vi "SEW.vi"() -> ()   [LabVIEW 2018]
uses:
  <userlib>/PNIO/PNIO.dll
panel:
  in  "Acknowledge":bool
  out "data_write":u8[](array[numeric])
  out "Status":u16 format="%x"
  out "Cluster":T1
  out "NIST_A":u32
  out "ZSW1":u16 format="%x"
  in  "ON/OFF":bool
  in  "Speed setpoint":sgl format="%.2f rpm"
  in  "stop":bool
  out "data_read":u8[](array[numeric]) format="%x"
  in  "number_bytes":u32=32
  out "error_write":u32 format="%x"
  out "error_read":u32 format="%x"
  out "state":bool
  in  "output_adress":u32
  in  "input_adress":u32
  out "ErrorCode":u32
  in  "Path":path=path "C:/Users/Messknecht/Desktop/LabVIEW/sew_eurodrive/SEW_Vi/PROFINET Driver_1.PROFINET Driver.PNDriverConfiguration.xml"
  in  "mac_adress":string="f8:b1:56:9d:5d:4b"
  out "function return":u32 format="%x"
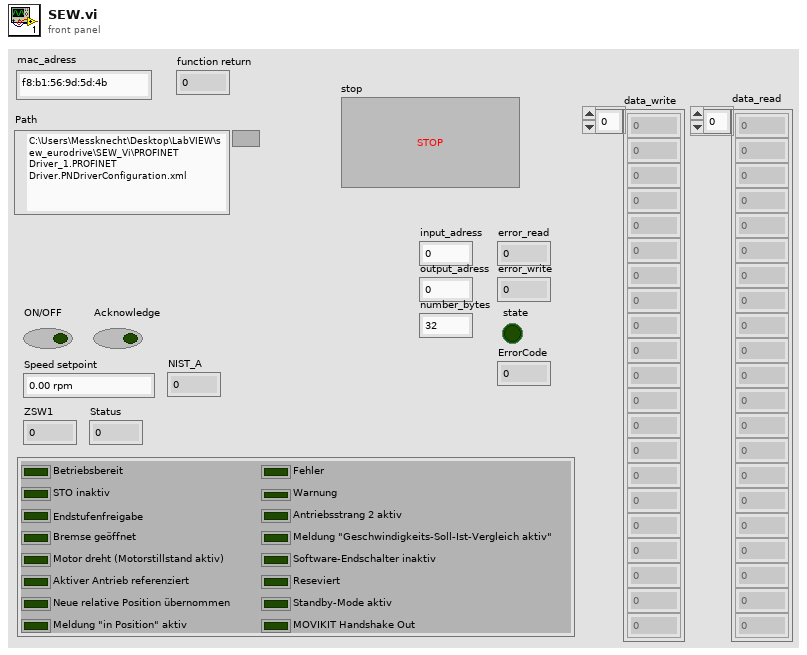
[diagram p1: front panel]
types:
  T1 = cluster{"Betriebsbereit":bool, "STO inaktiv":bool, "Endstufenfreigabe":bool, "Bremse geöffnet":bool, "Motor dreht (Motorstillstand aktiv)":bool, "Aktiver Antrieb referenziert":bool, "Neue relative Position übernommen":bool, "Meldung \"in Position\" aktiv":bool, "Fehler":bool, "Warnung":bool, "Antriebsstrang 2 aktiv":bool, "Meldung \"Geschwindigkeits-Soll-Ist-Vergleich aktiv\"":bool, "Software-Endschalter inaktiv":bool, "Reseviert":bool, "Standby-Mode aktiv":bool, "MOVIKIT Handshake Out":bool}
  T2 = cluster{"Boolean array[0]":bool, "Boolean array[1]":bool, "Boolean array[2]":bool, "Boolean array[3]":bool, "Boolean array[4]":bool, "Boolean array[5]":bool, "Boolean array[6]":bool, "Boolean array[7]":bool, "Boolean array[8]":bool, "Boolean array[9]":bool, "Boolean array[10]":bool, "Boolean array[11]":bool, "Boolean array[12]":bool, "Boolean array[13]":bool, "Boolean array[14]":bool, "Boolean array[15]":bool}
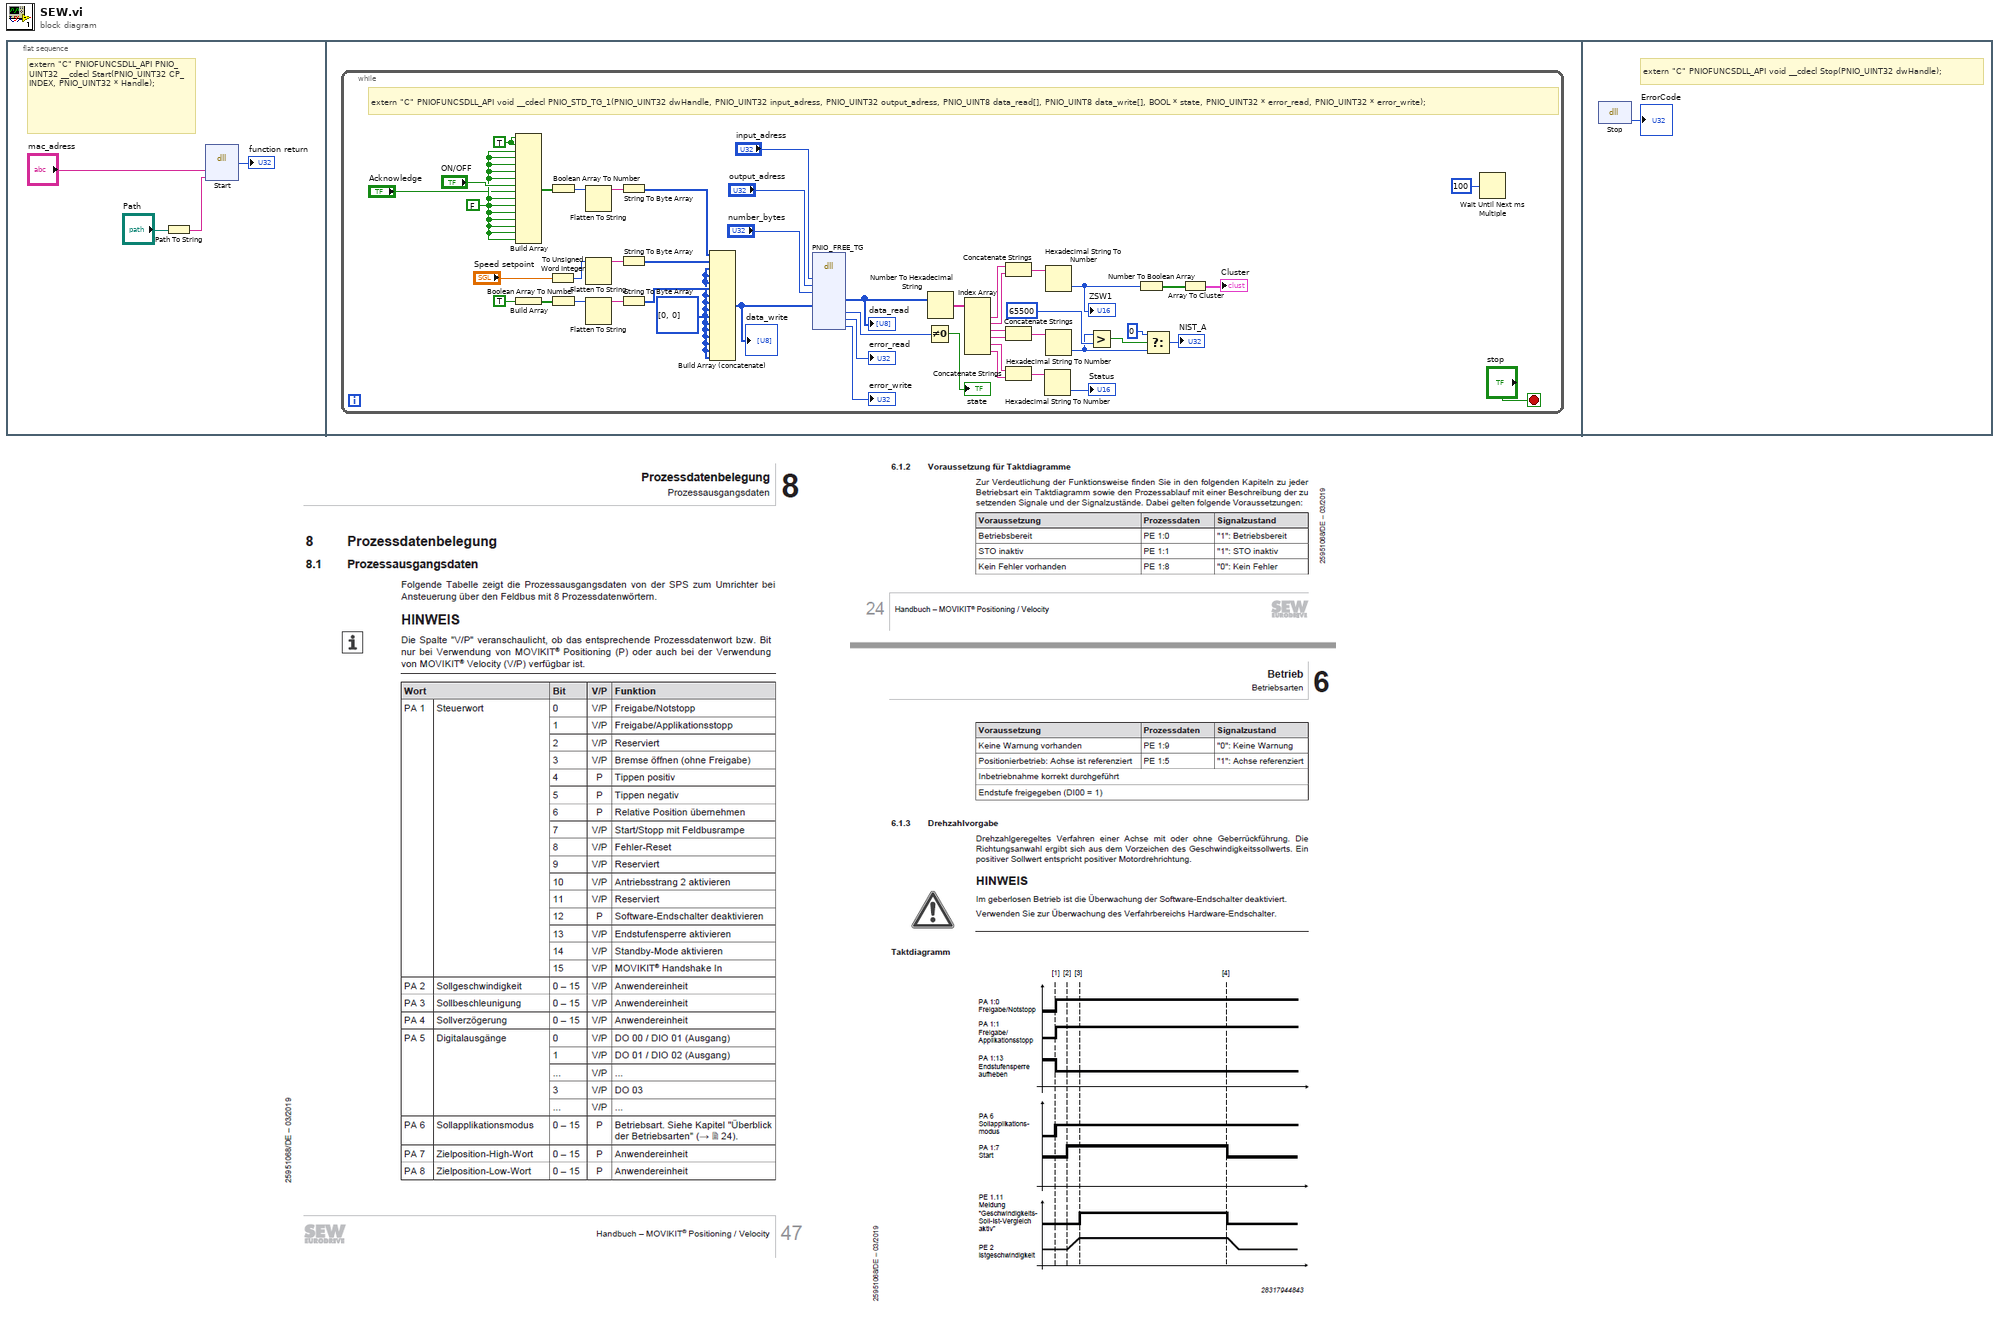
[diagram p0: block diagram]
diagram:
  n1 = flat-sequence {
    frame #0 {
      # "extern \"C\" PNIOFUNCSDLL_API PNIO_UINT32 __cdecl Start(PNIO_UINT32 CP_INDEX, PNIO_UINT32 * Handle);"
      n2 = Path To String(path="Path") -> (string=w1:string)
      n3 = dll-call lib="C:/Program Files (x86)/National Instruments/LabVIEW 2018/user.lib/PNIO/PNIO.dll" fn="Start"("mac_adress"="mac_adress", "xml_name"=w1) -> ("Rückgabetyp"=→"function return":u32)  [unwired: 5 in, 2 out]
    }
    frame #1 {
      n4 = while {
        stop <- "stop" stop-if-true
        w29 = u8[] [0, 0] ("unsigned byte array")
        w27 = FALSE
        w40 = TRUE
        # "extern \"C\" PNIOFUNCSDLL_API void __cdecl PNIO_STD_TG_1(PNIO_UINT32 dwHandle, PNIO_UINT32 input_adress, PNIO_UINT32 output_adress, PNIO_UINT8 data_read[], PNIO_UINT8 data_write[], BOOL * state, PNIO_UINT32 * error_read, PNIO_UINT32 * error_write);"
        n5 = Build Array(w40, w40, w27, w27, w27, w27, w27, "ON/OFF", "Acknowledge", w27, w27, w27, w27, w27, w27, w27) -> (w30:bool[])
        n6 = Build Array(TRUE) -> (w32:bool[])
        n7 = To Unsigned Word Integer(number="Speed setpoint") -> (unsigned 16bit integer=w39:u16)
        n8 = Boolean Array To Number ("Boolesches Array nach Zahl")(Boolean array=w30) -> (number=w41:u16)
        n9 = Boolean Array To Number ("Boolesches Array nach Zahl")(Boolean array=w32) -> (number=w33:u16)
        n10 = Flatten To String(anything=w41) -> (data string=w43:string)  [unwired: 3 in, 2 out]
        n11 = Flatten To String(anything=w39) -> (data string=w44:string)  [unwired: 3 in, 2 out]
        n12 = Flatten To String(anything=w33) -> (data string=w38:string)  [unwired: 3 in, 2 out]
        n13 = String To Byte Array(string=w43) -> (unsigned byte array=w42:u8[])
        n14 = String To Byte Array(string=w44) -> (unsigned byte array=w34:u8[])
        n15 = String To Byte Array(string=w38) -> (unsigned byte array=w37:u8[])
        n16 = Build Array (concatenate)(w42, w34, w29, w29, w29, w37, w29, w29, w29, w29, w29, w29, w29, w29, w29, w29) -> (w35:u8[])
        "data_write" <- w35
        n17 = dll-call lib="C:/Program Files (x86)/National Instruments/LabVIEW 2018/user.lib/PNIO/PNIO.*" fn="PNIO_FREE_TG"("input_adress"="input_adress", "output_adress"="output_adress", "number_bytes"="number_bytes", "data_write"=w35) -> ("data_read"=w25:u8[], "state"=w48:i32, "error_read"=→"error_read":u32, "error_write"=→"error_write":u32)  [unwired: 12 in, 2 out]
        "data_read" <- w25
        n18 = Not Equal To 0?(x=w48) -> (x != 0?=→"state":bool)
        n19 = Number To Hexadecimal String(2:w25) -> (0:w24:string[])  [unwired: 1 in]
        n20 = Index Array(array=w24) -> (element #1=w21:string, element #2=w20:string, element #3=w18:string, element #4=w17:string, element #5=w13:string, element #6=w12:string)  [unwired: 6 in]
        n21 = Concatenate Strings(w21, w20) -> (w19:string)
        n22 = Concatenate Strings(w18, w17) -> (w16:string)
        n23 = Concatenate Strings(w13, w12) -> (w15:string)
        n24 = Hexadecimal String To Number(string=w15) -> (number=→"Status":u32)  [unwired: 2 in, 1 out]
        n25 = Hexadecimal String To Number(string=w19) -> (number=w11:u32)  [unwired: 2 in, 1 out]
        "ZSW1" <- w11
        n26 = Hexadecimal String To Number(string=w16) -> (number=w7:u32)  [unwired: 2 in, 1 out]
        n27 = Greater?(x=w7, y=65500) -> (0:w9:bool)
        n28 = Number To Boolean Array(number=w11) -> (Boolean array=w23:bool[])
        n29 = Select(t=0, s=w9, f=w7) -> (s? t:f=→"NIST_A":u32)
        n30 = Array To Cluster(array=w23) -> (cluster=→"Cluster":T2)
        n31 = Wait Until Next ms Multiple(millisecond multiple=u32 100) -> ()  [unwired: 1 out]
      }
    }
    frame #2 {
      # "extern \"C\" PNIOFUNCSDLL_API void __cdecl Stop(PNIO_UINT32 dwHandle);"
      n32 = dll-call lib="C:/Program Files (x86)/National Instruments/LabVIEW 2018/user.lib/PNIO/PNIO.dll" fn="Stop"() -> ("ErrorCode"=→"ErrorCode":i32)  [unwired: 3 in, 2 out]
    }
  }
